vi "Draw.vi"(8 "error in (no error)":errorcluster, 10 "picture in (empty picture)":picture, 11 "Picture in":refnum<class "Picture.lvclass">) -> (0 "error out":errorcluster, 2 "picture out":picture, 3 "Picture out":refnum<class "Picture.lvclass">)   [LabVIEW 2020, in "Picture.lvclass"]
doc: "Draw a picture"
uses:
  Picture.lvclass
  Picture.lvclass/Picture.ctl
  Graphics Object/Graphics Object.lvclass
panel:
  # "expressionflow.com"
  # "Copyright (c) 2008 Tomi Maila. All rights reserved."
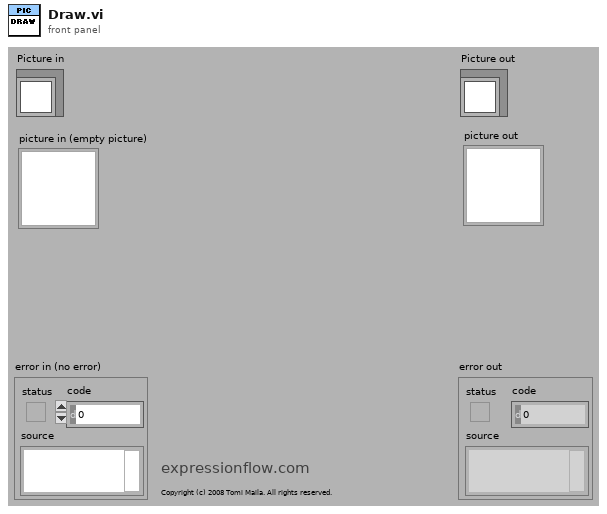
[diagram p1: front panel]
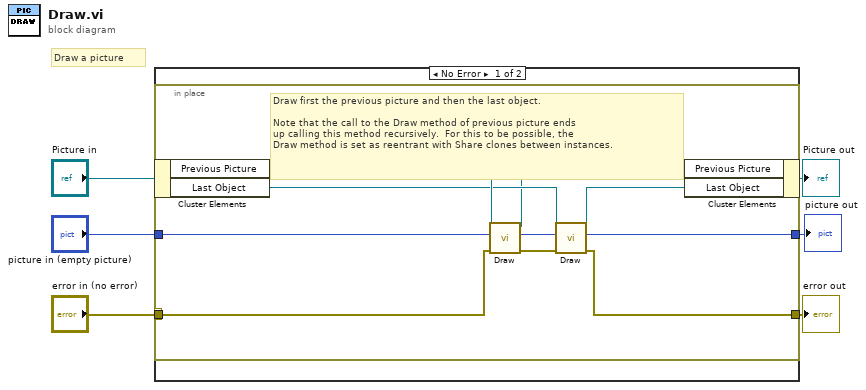
[diagram p0: block diagram]
diagram:
  # "Draw a picture"
  n1 = case shown="No Error" "error in (no error)" {
    selector: "error in (no error)" -> [w8 w25]
    tunnel: [w9 w25] -> w5
    tunnel: [w7 w24] -> w3
    tunnel: "Picture in" -> [w11 w24]
    tunnel: "picture in (empty picture)" -> [w12 w23]
    tunnel: [w10 w23] -> w1
    frame No Error {
      n2 = in-place {
        in-place-border: w12 -> [w22]
        in-place-border: [w16] -> w10
        in-place-border: [w15] -> w9
        in-place-border: w8 -> [w13]
        # "Draw first the previous picture and then the last object. \n\nNote that the call to the Draw method of previous picture ends\nup calling this method recursively.  For this to be possible, the \nDraw method is set as reentrant with Share clones between instances."
        n3 = in-place-cluster #1(w11) -> ("Previous Picture"=w21:refnum<class "Graphics Object.lvclass">, "Last Object"=w20:refnum<class "Graphics Object.lvclass">)
        n4 = call-dynamic "Draw.vi"("error in (no error)"=w13, "picture in (empty picture)"=w22, "Geometric Object in"=w21) -> ("error out"=w14:errorcluster, "picture out"=w19:picture, "Geometric Object out"=w18:refnum<class "Graphics Object.lvclass">)  [unwired: 6 in]
        n5 = call-dynamic "Draw.vi"("error in (no error)"=w14, "picture in (empty picture)"=w19, "Geometric Object in"=w20) -> ("error out"=w15:errorcluster, "picture out"=w16:picture, "Geometric Object out"=w17:refnum<class "Graphics Object.lvclass">)  [unwired: 6 in]
        n6 = in-place-cluster #1("Previous Picture"=w18, "Last Object"=w17) -> (w7:refnum<class "Picture.lvclass">)
      }
    }
    frame Error {
    }
  }
  "error out" <- w5
  "Picture out" <- w3
  "picture out" <- w1
